vi "Get Center Location.vi"(0 "GMap Control Ref":refnum<k24>, 11 "error in (no error)":errorcluster) -> (4 "GMap Control Ref Out":refnum<k24>, 6 "Lat":dbl, 8 "Lng":dbl, 10 "LocationMiddle":refnum<k24>, 15 "error out":errorcluster)   [LabVIEW 2014]
uses:
  C:/Robotic_Systems/Products/Surveyor/Software/Ground Station/Data/Mapping DLL/GMap.NET.WindowsForms.dll
  Data/Mapping DLL/GMap.NET.WindowsForms.dll
  C:/Robotic_Systems/Products/Surveyor/Software/Ground Station/Data/Mapping DLL/GMap.NET.Core.dll
  Data/Mapping DLL/GMap.NET.Core.dll
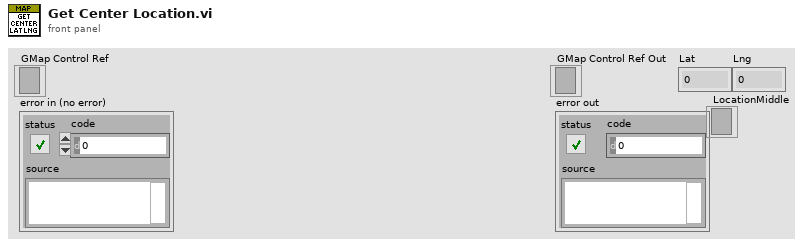
[diagram p1: front panel]
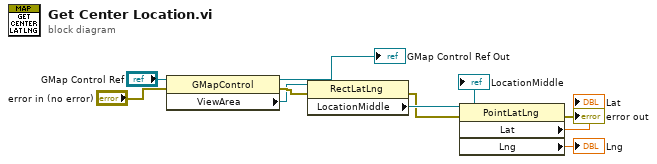
[diagram p0: block diagram]
diagram:
  n1 = property class="GMapControl"(reference="GMap Control Ref", error in="error in (no error)") -> (reference out=→"GMap Control Ref Out":refnum<k24>, error out=w9:errorcluster, "ViewArea"=w1:refnum<k24>)
  n2 = property class="RectLatLng"(reference=w1, error in=w9) -> (error out=w8:errorcluster, "LocationMiddle"=w10:refnum<k24>)  [unwired: 1 out]
  "LocationMiddle" <- w10
  n3 = property class="PointLatLng"(reference=w10, error in=w8) -> (error out=→"error out":errorcluster, "Lat"=→"Lat":dbl, "Lng"=→"Lng":dbl)  [unwired: 1 out]
